vi "ni579x Route Signal.vi"(0 "Register Bus":T1, 1 "source":string(combo)="None", 7 "destination":string(combo)="Rx Mixer Input", 11 "Error In":errorcluster) -> (4 "Register Bus (out)":T1, 15 "Error Out":errorcluster)   [LabVIEW 2015, in "ni579x Config v2 Host.lvlib"]
doc: "Routes a signal in the FAM from the specified source to the specified destination terminal.\n\n<B>Input Parameters</B>\n\n<B>Register Bus</B> The Register Bus object created by the ni579x Open VI and used as the session handle for the NI-579x Configuration Design Library.\n\n<B>source</B> The source signal.\n\"None\"- disconnect route to destination.\n\"LO1\"- the local oscillator.\n\"LO In\" the LO IN front-panel terminal.\n\"Rx In\"- the RX IN front-panel terminal.\n\"Tx Mixer Output\"- the output of the Tx Mixer\n\"Tx I (Mixer Bypass)\"- the I component of the baseband Tx signal, bypassing the Tx Mixer\n\"Sample Clock\"\n\"Reference Clock\"- the signal used as the reference clock for the Sample Clock and LO\n\n<B>destination</B> The destination terminal.\n\"Rx Mixer Input\"- the modulation signal input to the Rx Mixer\n\"Rx Mixer LO Input\"- the LO signal input to the Rx Mixer\n\"Tx Mixer LO Input\"- the LO signal input to the Tx Mixer\n\"Tx Out\"- the TX OUT front-panel terminal\n\"LO Out\"- the LO OUT front-panel terminal\n\"Clk Out\"- the CLK OUT front-panel terminal\n\n<B>Output Parameters</B>\n\n<B>Register Bus (out)</B> The Register Bus object created by the ni579x Open VI and used as the session handle for the NI-579x Configuration Design Library."
uses:
  <instrlib>/ni579x/Config/v2/Host/ni579x Config v2 Host.lvlib
  <instrlib>/_niInstr/Register Bus/v0/Host/Public/Register Bus Session.ctl
  <instrlib>/_niInstr/Register Bus/v0/Host/Private/Session Data.ctl
  <instrlib>/ni579x/Config/v2/Shared/Types/ni579x Route Signal Source Enum.ctl
  <instrlib>/ni579x/Config/v2/Shared/Types/ni579x Route Signal Destination Enum.ctl
  <instrlib>/ni579x/Config/v2/Shared/Types/ni579x Routing Mux Configuration.ctl
  <instrlib>/ni579x/Config/v2/Shared/Types/ni579x Routing Mux.ctl
  <instrlib>/ni579x/Config/v2/Shared/Types/ni579x User Command.ctl
  <instrlib>/ni579x/Config/v2/Shared/Types/ni579x User Command ID.ctl
  <instrlib>/ni579x/Config/v2/Shared/ni579x Config v2 Shared.lvlib
  <instrlib>/_niInstr/Register Bus/v0/Host/niInstr Register Bus v0 Host.lvlib
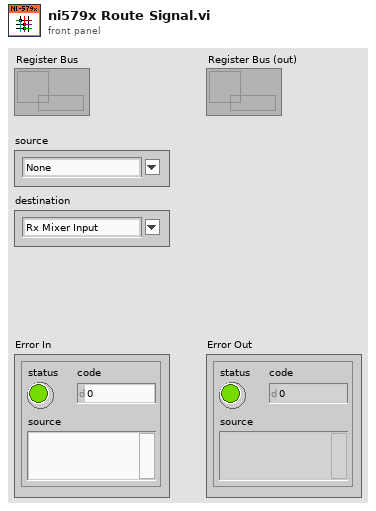
[diagram p1: front panel]
types:
  T1 = typedef "niInstr Register Bus v0 Host.lvlib/Register Bus Session.ctl" = refnum<queue>
  T2 = typedef "ni579x Config v2 Shared.lvlib/ni579x Route Signal Source Enum.ctl" = enum16{"None", "LO1", "LO2", "LO In", "Rx In", "Tx Mixer Output", "Tx I", "Sample Clock", "Reference Clock", "Invalid"}
  T3 = typedef "ni579x Config v2 Shared.lvlib/ni579x Route Signal Destination Enum.ctl" = enum16{"Rx Mixer Input", "Rx Mixer LO Input", "Tx Mixer LO Input", "Tx Out", "LO Out", "Clk Out", "Invalid"}
  T4 = typedef "ni579x Config v2 Shared.lvlib/ni579x User Command.ctl" = cluster{"User Data 0":u8, "User Data 1":u8, "User Command ID":T5}
  T5 = typedef "ni579x Config v2 Shared.lvlib/ni579x User Command ID.ctl" = u8
  T6 = typedef "ni579x Config v2 Shared.lvlib/ni579x Routing Mux Configuration.ctl" = cluster{"Routing Mux":T7, "Mux Setting":u8}
  T7 = typedef "ni579x Config v2 Shared.lvlib/ni579x Routing Mux.ctl" = enum8{"Rx Mixer LO Input", "Tx Mixer LO Input", "LO Out", "Tx Mixer Bypass", "Rx Mixer Input", "Tx Path", "Rx Cal"}
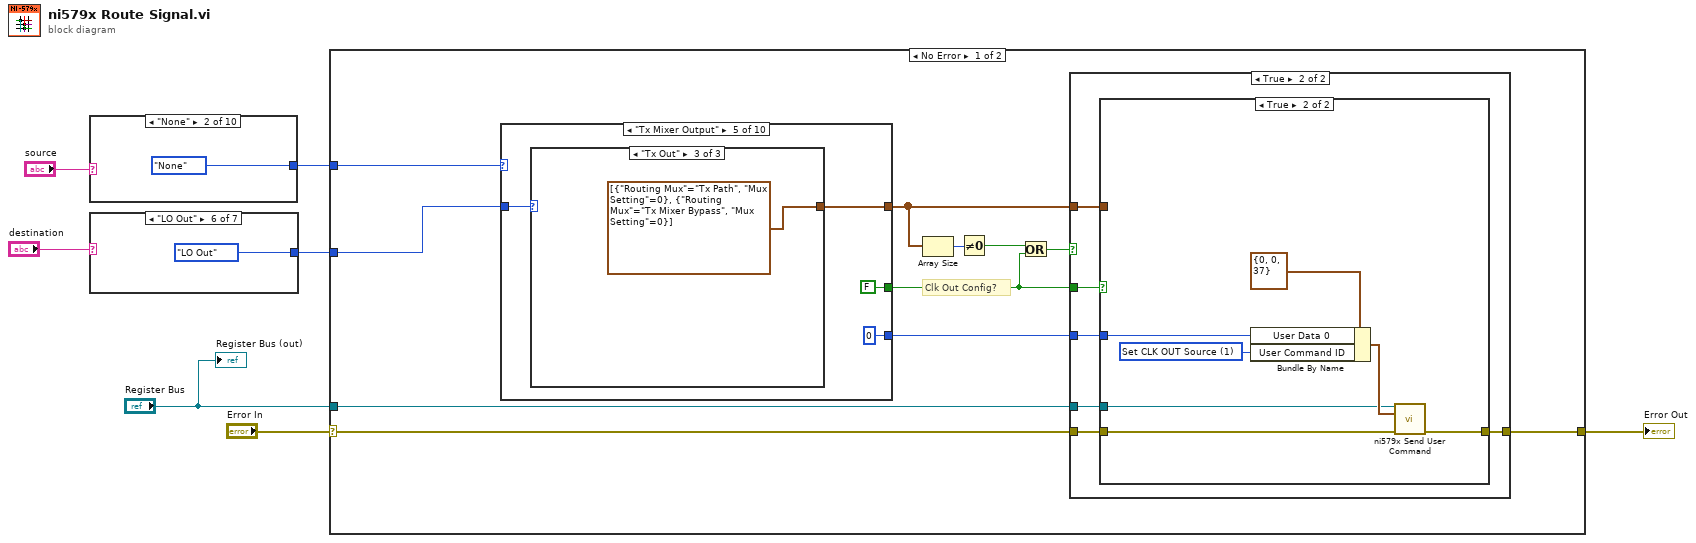
[diagram p0: block diagram]
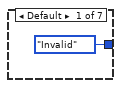
[diagram p2: hidden frame]
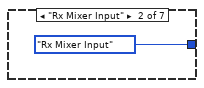
[diagram p3: hidden frame]
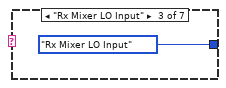
[diagram p4: hidden frame]
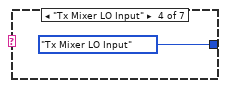
[diagram p5: hidden frame]
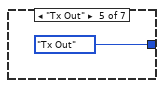
[diagram p6: hidden frame]
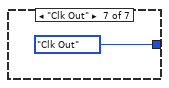
[diagram p7: hidden frame]
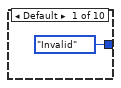
[diagram p8: hidden frame]
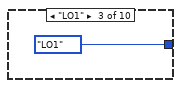
[diagram p9: hidden frame]
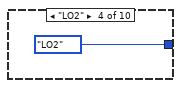
[diagram p10: hidden frame]
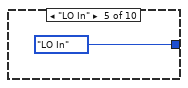
[diagram p11: hidden frame]
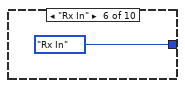
[diagram p12: hidden frame]
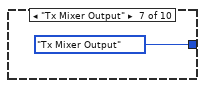
[diagram p13: hidden frame]
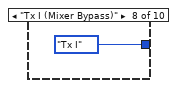
[diagram p14: hidden frame]
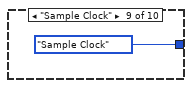
[diagram p15: hidden frame]
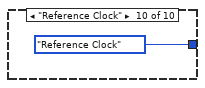
[diagram p16: hidden frame]
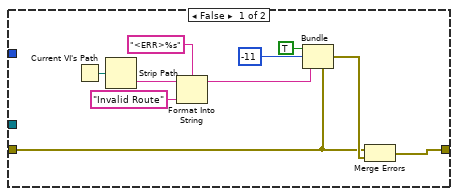
[diagram p17: hidden frame]
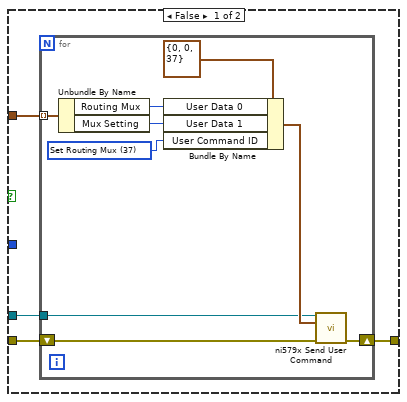
[diagram p18: hidden frame]
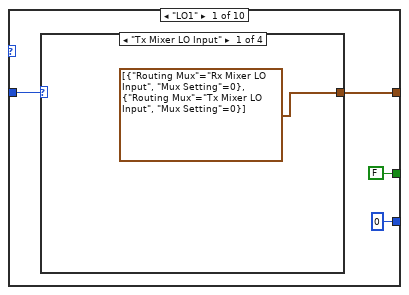
[diagram p19: hidden frame]
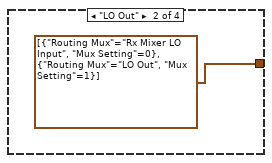
[diagram p20: hidden frame]
diagram:
  n1 = case shown="\"None\"" "source" {
    tunnel: [ni579x_Route_Signal_Source_Enum."Invalid" ("source") ni579x_Route_Signal_Source_Enum."None" ("source") ni579x_Route_Signal_Source_Enum."LO1" ("source") ni579x_Route_Signal_Source_Enum."LO2" ("source") ni579x_Route_Signal_Source_Enum."LO In" ("source") ni579x_Route_Signal_Source_Enum."Rx In" ("source") ni579x_Route_Signal_Source_Enum."Tx Mixer Output" ("source") ni579x_Route_Signal_Source_Enum."Tx I" ("source") ni579x_Route_Signal_Source_Enum."Sample Clock" ("source") ni579x_Route_Signal_Source_Enum."Reference Clock" ("source")] -> w3
    frame Default {
    }
    frame "None" {
    }
    frame "LO1" {
    }
    frame "LO2" {
    }
    frame "LO In" {
    }
    frame "Rx In" {
    }
    frame "Tx Mixer Output" {
    }
    frame "Tx I (Mixer Bypass)" {
    }
    frame "Sample Clock" {
    }
    frame "Reference Clock" {
    }
  }
  n2 = case shown="\"LO Out\"" "destination" {
    tunnel: [ni579x_Route_Signal_Destination_Enum."Invalid" ("destination") ni579x_Route_Signal_Destination_Enum."Rx Mixer Input" ("destination") ni579x_Route_Signal_Destination_Enum."Rx Mixer LO Input" ("destination") ni579x_Route_Signal_Destination_Enum."Tx Mixer LO Input" ("destination") ni579x_Route_Signal_Destination_Enum."Tx Out" ("destination") ni579x_Route_Signal_Destination_Enum."LO Out" ("destination") ni579x_Route_Signal_Destination_Enum."Clk Out" ("destination")] -> w1
    frame Default {
    }
    frame "Rx Mixer Input" {
    }
    frame "Rx Mixer LO Input" {
    }
    frame "Tx Mixer LO Input" {
    }
    frame "Tx Out" {
    }
    frame "LO Out" {
    }
    frame "Clk Out" {
    }
  }
  n3 = case shown="No Error" "Error In" {
    selector: "Error In" -> [w33 w147]
    tunnel: [w31 w147] -> w6
    tunnel: "Register Bus" -> [w32 _]
    tunnel: w3 -> [w26 _]
    tunnel: w1 -> [w25 _]
    frame No Error {
      # "Clk Out Config?"
      n4 = case shown="\"Tx Mixer Output\"" w26 {
        tunnel: w25 -> [w75 w83 w91 w98 w104 w111 w118 w131 w139 _]
        tunnel: [w74 w82 w90 w97 w103 w110 w117 T6[] [] T6[] [] T6[] []] -> w35
        tunnel: [FALSE FALSE FALSE FALSE FALSE FALSE w116 w129 w137 FALSE] -> w28
        tunnel: [u8 0 u8 0 u8 0 u8 0 u8 0 u8 0 w115 w128 w136 u8 0] -> w27
        frame "LO1" {
          n5 = case shown="\"Tx Mixer LO Input\"" w75 {
            tunnel: [T6[] [{"Routing Mux"=enum."Rx Mixer LO Input", "Mux Setting"=0}, {"Routing Mux"=enum."Tx Mixer LO Input", "Mux Setting"=0}] T6[] [{"Routing Mux"=enum."Rx Mixer LO Input", "Mux Setting"=0}, {"Routing Mux"=enum."LO Out", "Mux Setting"=1}] T6[] [] T6[] [{"Routing Mux"=enum."Rx Mixer LO Input", "Mux Setting"=0}]] -> w74
            frame "Tx Mixer LO Input" {
            }
            frame "LO Out" {
            }
            frame Default {
            }
            frame "Rx Mixer LO Input" {
            }
          }
        }
        frame "LO In" {
          n6 = case shown="Default" w83 {
            tunnel: [T6[] [{"Routing Mux"=enum."Rx Mixer LO Input", "Mux Setting"=1}, {"Routing Mux"=enum."Tx Mixer LO Input", "Mux Setting"=0}] T6[] [{"Routing Mux"=enum."Rx Mixer LO Input", "Mux Setting"=1}, {"Routing Mux"=enum."LO Out", "Mux Setting"=1}] T6[] [] T6[] [{"Routing Mux"=enum."Rx Mixer LO Input", "Mux Setting"=1}]] -> w82
            frame "Tx Mixer LO Input" {
            }
            frame "LO Out" {
            }
            frame Default {
            }
            frame "Rx Mixer LO Input" {
            }
          }
        }
        frame "LO2" {
          n7 = case shown="Default" w91 {
            tunnel: [T6[] [{"Routing Mux"=enum."Tx Mixer LO Input", "Mux Setting"=1}] T6[] [] T6[] [{"Routing Mux"=enum."Rx Mixer Input", "Mux Setting"=1}, {"Routing Mux"=enum."Rx Cal", "Mux Setting"=1}]] -> w90
            frame "Tx Mixer LO Input" {
            }
            frame Default {
            }
            frame "Rx Mixer Input" {
            }
          }
        }
        frame "Rx In" {
          n8 = case shown="\"Rx Mixer Input\"" w98 {
            tunnel: [T6[] [] T6[] [{"Routing Mux"=enum."Rx Mixer Input", "Mux Setting"=0}]] -> w97
            frame Default {
            }
            frame "Rx Mixer Input" {
            }
          }
        }
        frame "Tx Mixer Output" {
          n9 = case shown="\"Tx Out\"" w104 {
            tunnel: [T6[] [] T6[] [{"Routing Mux"=enum."Rx Mixer Input", "Mux Setting"=1}, {"Routing Mux"=enum."Rx Cal", "Mux Setting"=0}, {"Routing Mux"=enum."Tx Path", "Mux Setting"=1}, {"Routing Mux"=enum."Tx Mixer Bypass", "Mux Setting"=0}] T6[] [{"Routing Mux"=enum."Tx Path", "Mux Setting"=0}, {"Routing Mux"=enum."Tx Mixer Bypass", "Mux Setting"=0}]] -> w103
            frame Default {
            }
            frame "Rx Mixer Input" {
            }
            frame "Tx Out" {
            }
          }
        }
        frame "Tx I" {
          n10 = case shown="\"Rx Mixer Input\"" w111 {
            tunnel: [T6[] [] T6[] [{"Routing Mux"=enum."Rx Mixer Input", "Mux Setting"=1}, {"Routing Mux"=enum."Rx Cal", "Mux Setting"=0}, {"Routing Mux"=enum."Tx Path", "Mux Setting"=1}, {"Routing Mux"=enum."Tx Mixer Bypass", "Mux Setting"=1}] T6[] [{"Routing Mux"=enum."Tx Path", "Mux Setting"=0}, {"Routing Mux"=enum."Tx Mixer Bypass", "Mux Setting"=1}]] -> w110
            frame Default {
            }
            frame "Rx Mixer Input" {
            }
            frame "Tx Out" {
            }
          }
        }
        frame "None" {
          n11 = case shown="Default" w118 {
            tunnel: [T6[] [] T6[] [] T6[] [{"Routing Mux"=enum."LO Out", "Mux Setting"=0}]] -> w117
            tunnel: [TRUE FALSE FALSE] -> w116
            tunnel: [u8 0 u8 0 u8 0] -> w115
            frame "Clk Out" {
            }
            frame Default {
            }
            frame "LO Out" {
            }
          }
        }
        frame "Sample Clock" {
          n12 = case shown="\"Clk Out\"" w131 {
            tunnel: [FALSE TRUE] -> w129
            tunnel: [u8 0 u8 2] -> w128
            frame Default {
            }
            frame "Clk Out" {
            }
          }
        }
        frame "Reference Clock" {
          n13 = case shown="\"Clk Out\"" w139 {
            tunnel: [FALSE TRUE] -> w137
            tunnel: [u8 0 u8 1] -> w136
            frame Default {
            }
            frame "Clk Out" {
            }
          }
        }
        frame Default {
        }
      }
      n14 = Array Size(array=w35) -> (size(s)=w34:i32)
      n15 = Not Equal To 0?(x=w34) -> (x != 0?=w30:bool)
      n16 = Or(x=w30, y=w28) -> (x .or. y?=w29:bool)
      n17 = case shown="True" w29 {
        tunnel: w35 -> [_ w51]
        tunnel: w33 -> [w37 w50]
        tunnel: w32 -> [_ w49]
        tunnel: [w36 w48] -> w31
        tunnel: w28 -> [_ w47]
        tunnel: w27 -> [_ w46]
        frame False {
          n18 = Current VI's Path() -> (path=w39:path)
          n19 = Strip Path(path=w39) -> (name=w40:string)  [unwired: 1 out]
          n20 = Format Into String(format string="<ERR>%s", initial string=w40, "Invalid Route" ("input 1")) -> (resulting string=w41:string)  [unwired: 1 in, 1 out]
          n21 = Bundle(cluster=w37, "status"=TRUE, "code"=-11, "source"=w41) -> (w42:errorcluster)
          n22 = Merge Errors(w37, w42) -> (w36:errorcluster)
        }
        frame True {
          n23 = case shown="True" w47 {
            tunnel: w51 -> [w55 _]
            tunnel: w50 -> [w54 w69]
            tunnel: w49 -> [w53 w67]
            tunnel: [w52 w68] -> w48
            tunnel: w46 -> [_ w66]
            frame False {
              n24 = for {
                tunnel: w55 -> [w63] mode=indexing
                shift-right: [w58] -> w52
                shift-left: w54 -> [w59]
                tunnel: w53 -> [w57]
                w56 = T5 37 items=["Set Clock Select"=0, "Set CLK OUT Source"=1, "DAC Sync User Start"=2, "DAC Sync User End"=3, "Enable Baseband Amp"=5, "Set Rx Attenuation Pre-LNA"=7, "Set Rx Attenuation Post-LNA"=8, "Set Tx Attenuation"=9, "Set LO Filter"=32, "Set Front End Filter"=33, "Enable LO"=34, "Set Routing Mux"=37, "Read Current Rev Lower"=240, "Read Current Rev Upper"=241, "Read Oldest Compat Rev Lower"=242, "Read Oldest Compat Rev Upper"=243, "Re-Initialize"=255] ("User Command ID")
                n25 = Unbundle By Name(w63) -> ("Routing Mux"=w62:T7, "Mux Setting"=w61:u8)
                n26 = Bundle By Name(cluster=T4 {"User Data 0"=0, "User Data 1"=0, "User Command ID"=37} ("User Command"), "User Data 0"=w62, "User Data 1"=w61, "User Command ID"=w56) -> (w60:T4)
                n27 = call <instrlib>:"ni579x Send User Command.vi"("Register Bus"=w57, "User Command"=w60, "Error In"=w59) -> ("Error Out"=w58:errorcluster)  [unwired: 8 in, 4 out]
              }
            }
            frame True {
              w65 = T5 1 items=["Set Clock Select"=0, "Set CLK OUT Source"=1, "DAC Sync User Start"=2, "DAC Sync User End"=3, "Enable Baseband Amp"=5, "Set Rx Attenuation Pre-LNA"=7, "Set Rx Attenuation Post-LNA"=8, "Set Tx Attenuation"=9, "Set LO Filter"=32, "Set Front End Filter"=33, "Enable LO"=34, "Set Routing Mux"=37, "Read Current Rev Lower"=240, "Read Current Rev Upper"=241, "Read Oldest Compat Rev Lower"=242, "Read Oldest Compat Rev Upper"=243, "Re-Initialize"=255] ("User Command ID")
              n28 = Bundle By Name(cluster=T4 {"User Data 0"=0, "User Data 1"=0, "User Command ID"=37} ("User Command"), "User Data 0"=w66, "User Command ID"=w65) -> (w70:T4)
              n29 = call <instrlib>:"ni579x Send User Command.vi"("Register Bus"=w67, "User Command"=w70, "Error In"=w69) -> ("Error Out"=w68:errorcluster)  [unwired: 8 in, 4 out]
            }
          }
        }
      }
    }
    frame Error {
    }
  }
  "Error Out" <- w6
  "Register Bus (out)" <- "Register Bus"
